vi "createDefaultGoals.vi"(8 "error in (no error)":errorcluster, 10 "WhichMonth":refnum<class "WhichMonth.lvclass">, 11 "Database in":refnum<class "Account History.lvclass">) -> (0 "error out":errorcluster, 3 "Database out":refnum<class "Account History.lvclass">)   [LabVIEW 2018, in "Account History.lvclass"]
uses:
  Account History.lvclass
  WhichMonth/WhichMonth.lvclass
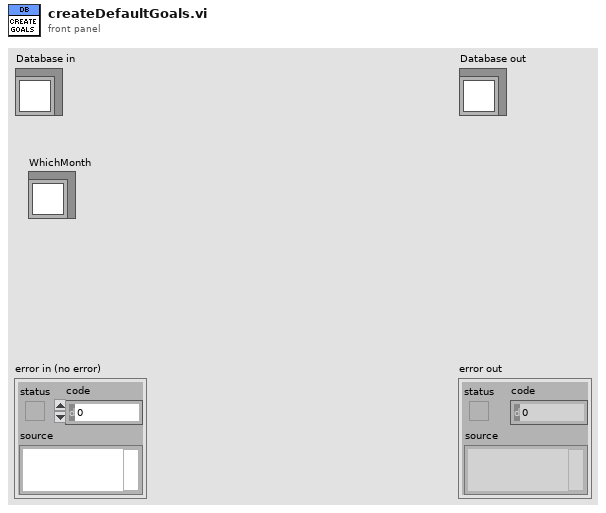
[diagram p1: front panel]
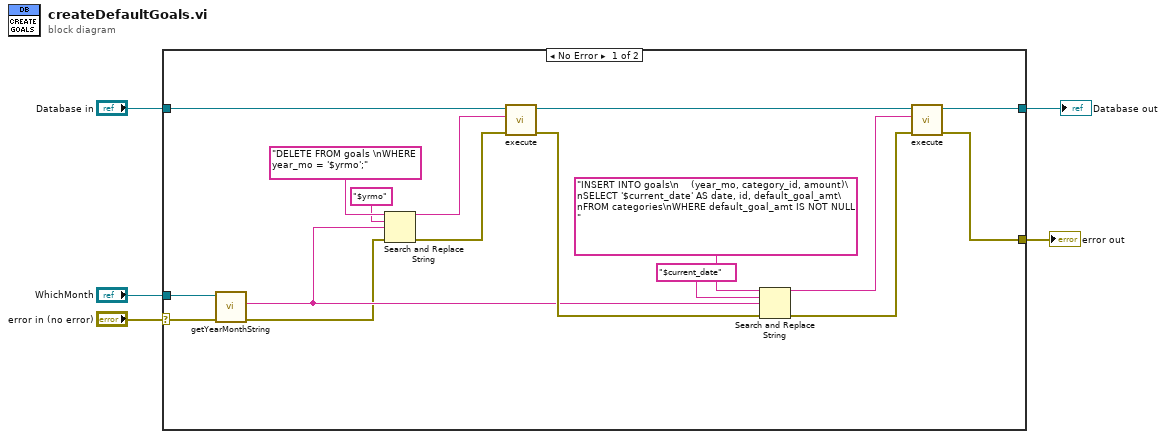
[diagram p0: block diagram]
diagram:
  n1 = case shown="No Error" "error in (no error)" {
    selector: "error in (no error)" -> [w7 w24]
    tunnel: [w20 w24] -> w4
    tunnel: [w21 w23] -> w2
    tunnel: "Database in" -> [w22 w23]
    tunnel: "WhichMonth" -> [w9 _]
    frame No Error {
      n2 = call "getYearMonthString.vi"("error in (no error)"=w7, "WhichMonth in"=w9) -> ("error out"=w6:errorcluster, "Year-Month"=w8:string)  [unwired: 7 in, 1 out]
      n3 = Search and Replace String(input string="DELETE FROM goals \nWHERE year_mo = '$yrmo';", search string="$yrmo", replace string=w8, error in=w6) -> (result string=w17:string, error out=w16:errorcluster)  [unwired: 4 in, 2 out]
      n4 = call "execute.vi"("error in (no error)"=w16, "SQL query"=w17, "Database in"=w22) -> ("error out"=w13:errorcluster, "Database out"=w15:refnum<class "Account History.lvclass">)  [unwired: 7 in]
      n5 = Search and Replace String(input string="INSERT INTO goals\n    (year_mo, category_id, amount)\nSELECT '$current_date' AS date, id, default_goal_amt\nFROM categories\nWHERE default_goal_amt IS NOT NULL  ", search string="$current_date", replace string=w8, error in=w13) -> (result string=w12:string, error out=w11:errorcluster)  [unwired: 4 in, 2 out]
      n6 = call "execute.vi"("error in (no error)"=w11, "SQL query"=w12, "Database in"=w15) -> ("error out"=w20:errorcluster, "Database out"=w21:refnum<class "Account History.lvclass">)  [unwired: 7 in]
    }
    frame Error {
    }
  }
  "error out" <- w4
  "Database out" <- w2
